vi "cal inst test.vi"() -> ()   [LabVIEW 2013]
uses:
  Libraries/California Instruments iX Series/California Instruments iX Series.lvlib
panel:
  in  "Enable Output (T: Enable)":bool
  in  "stop":bool
  in  "Tab Control":T1(tab)
  in  "Enable Current Protection (Enabled)":bool=TRUE
  in  "Current Level (0 A)":dbl
  in  "Current Protection Delay (0.1 Sec)":dbl=0.1
  in  "Voltage Mode (0: Fixed)":i32(ring) items=["Fixed", "Step", "Pulse", "List"]
  in  "Voltage Auto Level Control (0: On)":u16(ring) items=["On", "Off", "Regulation"]
  in  "Voltage Source (0:Internal)":u16(ring) items=["Internal", "External"]
  in  "Voltage Level (0V)":dbl
  in  "Transient Voltage Level (0V)":dbl
  in  "Voltage Protection Range (150V)":u16(ring)=150 items=["150"=150, "300"=300]
  in  "Voltage Limit (0.0 V)":dbl format="%.2g"
  in  "Phase (0°)":dbl
  in  "Triggered Phase (0°)":dbl
  in  "Phase Mode (0: Fixed)":i32(ring) items=["Fixed", "Step", "Pulse", "List"]
  in  "Frequency (60 Hz)":dbl=60.0
  in  "Triggered Frequency (60 Hz)":dbl=60.0
  in  "Frequency Mode (0: Fixed)":i32(ring) items=["Fixed", "Step", "Pulse", "List", "Sense", "External"]
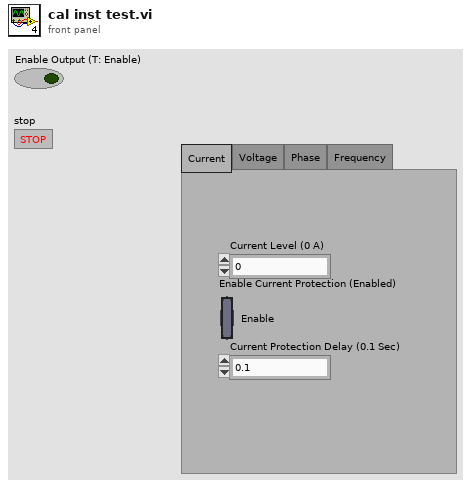
[diagram p1: front panel]
types:
  T1 = enum32{"Current", "Voltage", "Phase", "Frequency"}
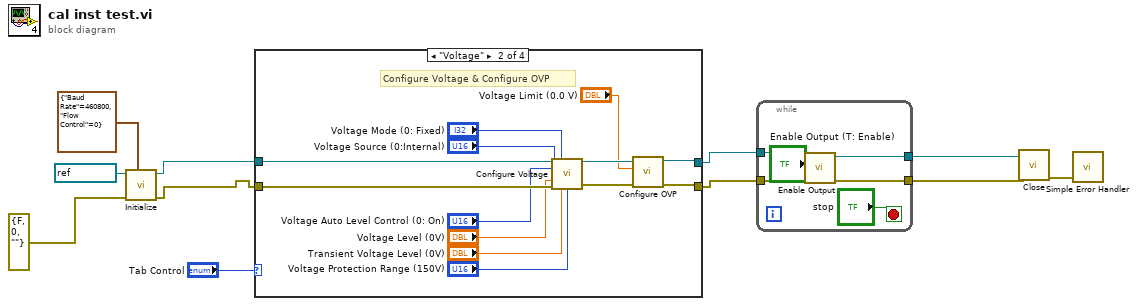
[diagram p0: block diagram]
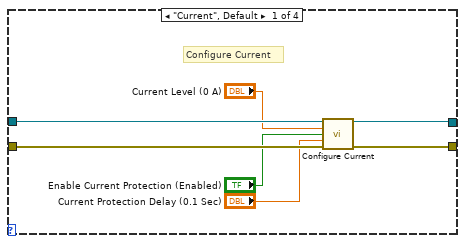
[diagram p2: hidden frame]
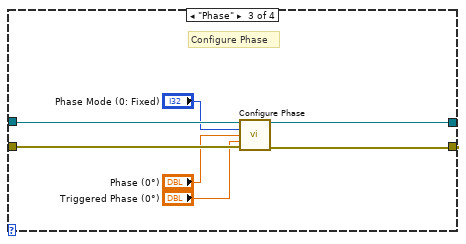
[diagram p3: hidden frame]
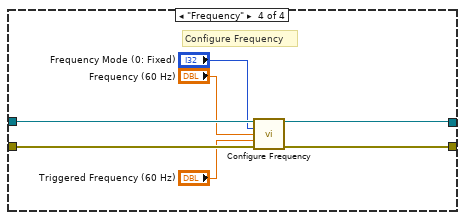
[diagram p4: hidden frame]
diagram:
  n1 = call "Initialize.vi"("Serial Configuration"=cluster{"Baud Rate":u32, "Flow Control":u16} {"Baud Rate"=460800, "Flow Control"=0}, "error in (no error)"=errorcluster {"status"=FALSE, "code"=0, "source"=""}, "VISA resource name"=refnum<visa-resource-name> "COM6") -> ("error out"=w5:errorcluster, "VISA resource name out"=w6:refnum<visa-resource-name>)  [unwired: 7 in]
  n2 = case shown="\"Voltage\"" "Tab Control" {
    tunnel: w6 -> [w18 w31 w38 w45]
    tunnel: w5 -> [w17 w30 w37 w44]
    tunnel: [w13 w20 w33 w40] -> w4
    tunnel: [w12 w19 w32 w39] -> w3
    frame "Current", Default {
      # "Configure Current"
      n3 = call "Configure Current.vi"("VISA resource name"=w18, "Current Level (0 A)"="Current Level (0 A)", "Enable Current Protection (Enabled)"="Enable Current Protection (Enabled)", "Current Protection Delay (0.1 Sec)"="Current Protection Delay (0.1 Sec)", "error in (no error)"=w17) -> ("VISA resource name out"=w13:refnum<visa-resource-name>, "error out"=w12:errorcluster)  [unwired: 9 in]
    }
    frame "Voltage" {
      # "Configure Voltage & Configure OVP"
      n4 = call "Configure Voltage.vi"("VISA resource name"=w31, "Voltage Mode (0: Fixed)"="Voltage Mode (0: Fixed)", "Voltage Auto Level Control (0: On)"="Voltage Auto Level Control (0: On)", "Voltage Source (0:Internal)"="Voltage Source (0:Internal)", "Voltage Level (0V)"="Voltage Level (0V)", "error in (no error)"=w30, "Transient Voltage Level (0V)"="Transient Voltage Level (0V)", "Voltage Protection Range (150V)"="Voltage Protection Range (150V)") -> ("VISA resource name out"=w23:refnum<visa-resource-name>, "error out"=w22:errorcluster)  [unwired: 6 in]
      n5 = call "Configure OVP.vi"("error in (no error)"=w22, "Voltage Limit (0.0 V)"="Voltage Limit (0.0 V)", "VISA resource name"=w23) -> ("error out"=w19:errorcluster, "VISA resource name out"=w20:refnum<visa-resource-name>)  [unwired: 7 in]
    }
    frame "Phase" {
      # "Configure Phase"
      n6 = call "Configure Phase.vi"("VISA resource name"=w38, "Phase Mode (0: Fixed)"="Phase Mode (0: Fixed)", "Phase (0°)"="Phase (0°)", "Triggered Phase (0°)"="Triggered Phase (0°)", "error in (no error)"=w37) -> ("VISA resource name out"=w33:refnum<visa-resource-name>, "error out"=w32:errorcluster)  [unwired: 9 in]
    }
    frame "Frequency" {
      # "Configure Frequency"
      n7 = call "Configure Frequency.vi"("VISA resource name"=w45, "Frequency Mode (0: Fixed)"="Frequency Mode (0: Fixed)", "Frequency (60 Hz)"="Frequency (60 Hz)", "Triggered Frequency (60 Hz)"="Triggered Frequency (60 Hz)", "error in (no error)"=w44) -> ("VISA resource name out"=w40:refnum<visa-resource-name>, "error out"=w39:errorcluster)  [unwired: 9 in]
    }
  }
  n8 = while {
    tunnel: w4 -> [w50]
    tunnel: w3 -> [w49]
    tunnel: [w48] -> w2
    tunnel: [w47] -> w1
    stop <- "stop" stop-if-true
    n9 = call "Enable Output.vi"("error in (no error)"=w49, "Enable Output (T: Enable)"="Enable Output (T: Enable)", "VISA resource name"=w50) -> ("error out"=w47:errorcluster, "VISA resource name out"=w48:refnum<visa-resource-name>)  [unwired: 7 in]
  }
  n10 = call "Close.vi"("error in (no error)"=w1, "VISA resource name"=w2) -> ("error out"=w8:errorcluster)  [unwired: 9 in]
  n11 = call <vilib>:"Simple Error Handler.vi"("error in (no error)"=w8) -> ()  [unwired: 4 in, 5 out]
